vi "PH_AxisGUI_NF2.set GUI elements.vi"(0 "i ref in":refnum<vi>, 5 "error in (no error)":errorcluster) -> (14 "i ref out":refnum<vi>, 19 "error out":errorcluster)   [LabVIEW 2014, in "PH_AxisGUI_NF2.lvlib"]
uses:
  PH_AxisGUI_NF2.lvlib
  PH_Basics/PH_Common/PH_Common.lvlib
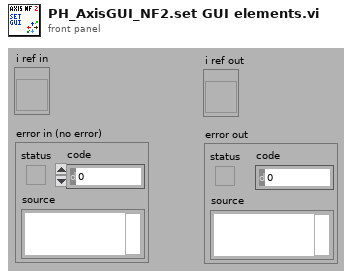
[diagram p1: front panel]
types:
  T1 = typedef "PH_AxisGUI_NF2.lvlib/PH_AxisGUI_NF2.i attribute.ctl" = cluster{"GUI Refs":cluster{"Delete":refnum<vi>, "Instance Status":refnum<vi>, "Width Axis 1":refnum<vi>, "Width Axis 2":refnum<vi>}, "Instance":string, "System":string, "Width Axis 1":i32, "Width Axis 2":i32, "Sign Change Axis 1":bool, "Sign Change Axis 2":bool, "Motor Axis 1":i32, "Motor Axis 2":i32}
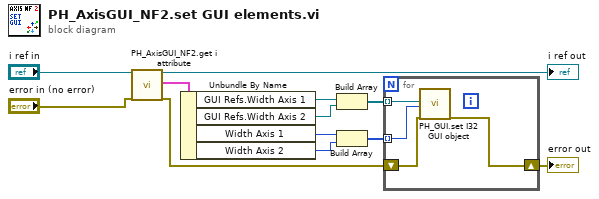
[diagram p0: block diagram]
diagram:
  n1 = call "PH_AxisGUI_NF2.get i attribute.vi"("i ref in"="i ref in", "error in (no error)"="error in (no error)") -> ("i ref out"=→"i ref out":refnum<vi>, "i attribute"=w9:T1, "error out"=w5:errorcluster)  [unwired: 15 in]
  n2 = Unbundle By Name(w9) -> ("GUI Refs.Width Axis 1"=w8:refnum<vi>, "GUI Refs.Width Axis 2"=w7:refnum<vi>, "Width Axis 1"=w3:i32, "Width Axis 2"=w2:i32)
  n3 = Build Array(w8, w7) -> (w6:refnum<vi>[])
  n4 = Build Array(w3, w2) -> (w1:i32[])
  n5 = for {
    tunnel: w6 -> [w16] mode=indexing
    shift-right: [w14] -> w4
    shift-left: w5 -> [w15]
    tunnel: w1 -> [w13] mode=indexing
    n6 = call "PH_GUI.set I32 GUI object.vi"("I32 GUI Ref"=w16, "value"=w13, "error in (no error)"=w15) -> ("error out"=w14:errorcluster)  [unwired: 16 in]
  }
  "error out" <- w4
